vi "Channel.Index.Set.vi"(8 "error in (no error)":errorcluster, 10 "Constants.Index":u16, 11 "Ref":T1 format="%.0x") -> (0 "error out":errorcluster, 3 "Ref out":T1 format="%.0x")   [LabVIEW 2019, in "Fuel Injector Analysis Addon System Explorer.lvlib"]
uses:
  Fuel Injector Analysis Addon System Explorer.lvlib
  <vilib>/NI VeriStand/Custom Device API/Custom Device Item Ref.ctl
  Addon Shared/SubVIs/Constants.vi
  <vilib>/NI VeriStand/Custom Device API/Set Item Property (U16).vi
  <vilib>/NI VeriStand/Custom Device API/Custom Device API.lvlib
  Addon Shared/Fuel Injector Analysis Addon Shared.lvlib
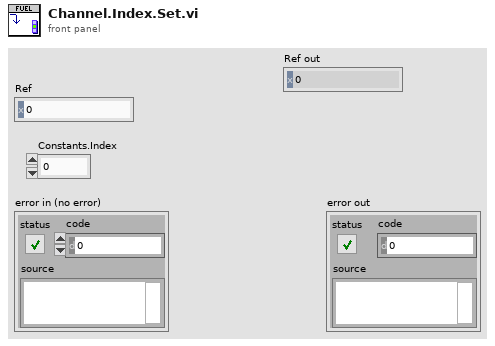
[diagram p1: front panel]
types:
  T1 = typedef "Custom Device API.lvlib/Custom Device Item Ref.ctl" = u64
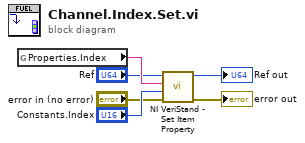
[diagram p0: block diagram]
diagram:
  n1 = global read "Constants.vi" "Properties.Index"() -> (w5:string)
  n2 = call-poly <vilib>:"NI VeriStand - Set Item Property.vi"("error in (no error)"="error in (no error)", "Value"="Constants.Index", "Property Name"=w5, "Item Ref in"="Ref") -> ("error out"=→"error out":errorcluster, "Item Ref out"=→"Ref out":T1)  [unwired: 5 in, 1 out]
